vi "Configure Multi Eval Meas Limit Inband Emission IQ Offset.vi"(6 "Offset 1 (-20.0)":dbl=-20.0 format="%^.3e", 7 "Offset 0 (-25.0)":dbl=-25.0 format="%^.3e", 8 "error in (no error)":errorcluster, 9 "Modulation (Pi/2-BPSK)":i32(ring) items=["Pi/2-BPSK", "QPSK", "16-QAM", "64-QAM", "256-QAM"], 10 "Instance (1)":T1=1, 11 "VISA resource name":refnum<visa-resource-name>) -> (0 "error out":errorcluster, 3 "VISA resource name out":refnum<visa-resource-name>)   [LabVIEW 2020, in "Rohde&Schwarz CMXP NR FR2 Measurement.lvlib"]
doc: "Defines I/Q origin offset values used for calculation of an upper limit for the inband emission. Two different values can be set for two TX power ranges.\n\nAttributes:\nRSCMXPNRFR2M_ATTR_MULTI_EVAL_MEASUREMENT_LIMIT_PHBPSK_INBAND_EMISSION_IQ_OFFSET\nRSCMXPNRFR2M_ATTR_MULTI_EVAL_MEASUREMENT_LIMIT_QPSK_INBAND_EMISSION_IQ_OFFSET\nRSCMXPNRFR2M_ATTR_MULTI_EVAL_MEASUREMENT_LIMIT_QAM16_INBAND_EMISSION_IQ_OFFSET\nRSCMXPNRFR2M_ATTR_MULTI_EVAL_MEASUREMENT_LIMIT_QAM64_INBAND_EMISSION_IQ_OFFSET\nRSCMXPNRFR2M_ATTR_MULTI_EVAL_MEASUREMENT_LIMIT_QAM256_INBAND_EMISSION_IQ_OFFSET\n\nRemote-control commands:\nCONFigure:NRMMw:MEAS<i>:MEValuation:LIMit:PHBPsk:IBE:IQOFfset\nCONFigure:NRMMw:MEAS<i>:MEValuation:LIMit:QPSK:IBE:IQOFfset\nCONFigure:NRMMw:MEAS<i>:MEValuation:LIMit:QAM<order>:IBE:IQOFfset"
uses:
  <instrlib>/Rohde&Schwarz CMXP NR FR2 Measurement/Rohde&Schwarz CMXP NR FR2 Measurement.lvlib
  <instrlib>/Rohde&Schwarz CMXP NR FR2 Measurement/Private/_Instance.ctl
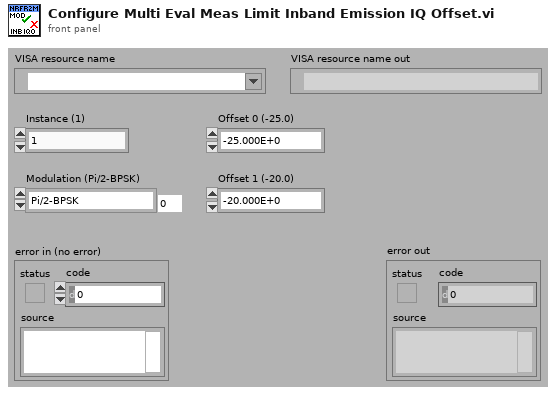
[diagram p1: front panel]
types:
  T1 = typedef "Rohde&Schwarz CMXP NR FR2 Measurement.lvlib/_Instance.ctl" = i32
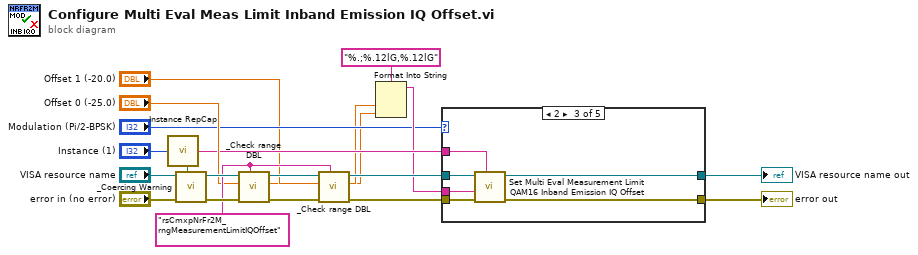
[diagram p0: block diagram]
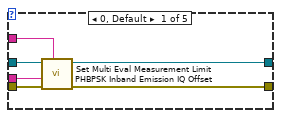
[diagram p2: hidden frame]
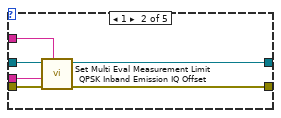
[diagram p3: hidden frame]
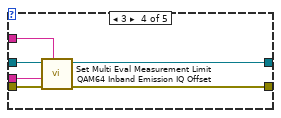
[diagram p4: hidden frame]
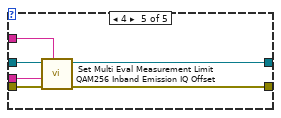
[diagram p5: hidden frame]
diagram:
  w16 = "rsCmxpNrFr2M_rngMeasurementLimitIQOffset"
  n1 = call <instrlib>:"Instance RepCap.vi"("Instance In"="Instance (1)") -> ("In Range?"=w19:bool, "RepCap Identifier Out"=w9:string)  [unwired: 1 in]
  n2 = call <instrlib>:"_Coercing Warning.vi"("In Range?"=w19, "error in (no error)"="error in (no error)", "VISA resource name"="VISA resource name") -> ("error out"=w18:errorcluster, "VISA resource name out"=w17:refnum<visa-resource-name>)  [unwired: 7 in]
  n3 = call <instrlib>:"_Check range DBL.vi"("Range Table Identifier"=w16, "error in (no error)"=w18, "DBL Value In"="Offset 0 (-25.0)", "VISA resource name"=w17) -> ("error out"=w14:errorcluster, "DBL Value Out"=w3:dbl, "VISA resource name out"=w13:refnum<visa-resource-name>)  [unwired: 5 in]
  n4 = call <instrlib>:"_Check range DBL.vi"("Range Table Identifier"=w16, "error in (no error)"=w14, "DBL Value In"="Offset 1 (-20.0)", "VISA resource name"=w13) -> ("error out"=w10:errorcluster, "DBL Value Out"=w2:dbl, "VISA resource name out"=w11:refnum<visa-resource-name>)  [unwired: 5 in]
  n5 = Format Into String(format string="%.;%.12lG,%.12lG", w3, w2) -> (resulting string=w8:string)  [unwired: 2 in, 1 out]
  n6 = case shown="2" "Modulation (Pi/2-BPSK)" {
    tunnel: w11 -> [w27 w33 w39 w45 w51]
    tunnel: w10 -> [w26 w32 w38 w44 w50]
    tunnel: w9 -> [w25 w31 w37 w43 w49]
    tunnel: w8 -> [w22 w28 w34 w40 w46]
    tunnel: [w24 w30 w36 w42 w48] -> w5
    tunnel: [w23 w29 w35 w41 w47] -> w6
    frame 0, Default {
      n7 = call "Set Multi Eval Measurement Limit PHBPSK Inband Emission IQ Offset"("Repeated Capabilities"=w25, "error in (no error)"=w26, "Multi Eval Measurement Limit PHBPSK Inband Emission IQ Offset ()"=w22, "instrument handle"=w27) -> ("error out"=w24:errorcluster, "instrument handle out"=w23:refnum<visa-resource-name>)  [unwired: 6 in]
    }
    frame 1 {
      n8 = call "Set Multi Eval Measurement Limit QPSK Inband Emission IQ Offset"("Repeated Capabilities"=w31, "error in (no error)"=w32, "Multi Eval Measurement Limit QPSK Inband Emission IQ Offset ()"=w28, "instrument handle"=w33) -> ("error out"=w30:errorcluster, "instrument handle out"=w29:refnum<visa-resource-name>)  [unwired: 6 in]
    }
    frame 2 {
      n9 = call "Set Multi Eval Measurement Limit QAM16 Inband Emission IQ Offset"("Repeated Capabilities"=w37, "error in (no error)"=w38, "Multi Eval Measurement Limit QAM16 Inband Emission IQ Offset ()"=w34, "instrument handle"=w39) -> ("error out"=w36:errorcluster, "instrument handle out"=w35:refnum<visa-resource-name>)  [unwired: 6 in]
    }
    frame 3 {
      n10 = call "Set Multi Eval Measurement Limit QAM64 Inband Emission IQ Offset"("Repeated Capabilities"=w43, "error in (no error)"=w44, "Multi Eval Measurement Limit QAM64 Inband Emission IQ Offset ()"=w40, "instrument handle"=w45) -> ("error out"=w42:errorcluster, "instrument handle out"=w41:refnum<visa-resource-name>)  [unwired: 6 in]
    }
    frame 4 {
      n11 = call "Set Multi Eval Measurement Limit QAM256 Inband Emission IQ Offset"("Repeated Capabilities"=w49, "error in (no error)"=w50, "Multi Eval Measurement Limit QAM256 Inband Emission IQ Offset ()"=w46, "instrument handle"=w51) -> ("error out"=w48:errorcluster, "instrument handle out"=w47:refnum<visa-resource-name>)  [unwired: 6 in]
    }
  }
  "error out" <- w5
  "VISA resource name out" <- w6
